vi "ATDome_cancelCallback_command_closeShutterackcmd.vi"(8 "error in (no error)":errorcluster) -> (0 "error out":errorcluster, 3 "function return":i32)   [LabVIEW 2016, in "SALLV_ATDome.lvlib"]
doc: "int ATDome_shm_cancelCallback_command_closeShutter_ackcmdLV();"
uses:
  SALLV_ATDome.lvlib
  SALLV_ATDome.so
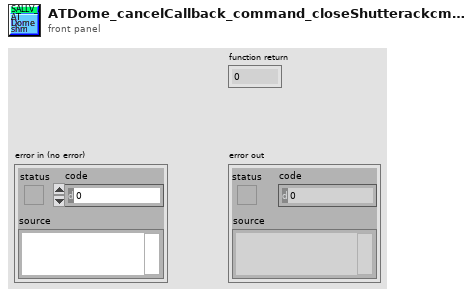
[diagram p1: front panel]
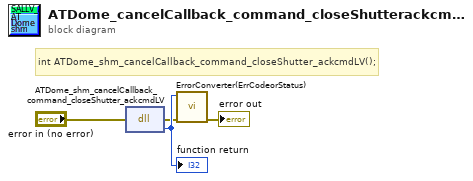
[diagram p0: block diagram]
diagram:
  # "int ATDome_shm_cancelCallback_command_closeShutter_ackcmdLV();"
  n1 = dll-call lib="home/andres/Desktop/SAL_ATDome/SALLV_ATDome.*" fn="ATDome_shm_cancelCallback_command_closeShutter_ackcmdLV"(error in="error in (no error)") -> (error out=w2:errorcluster, w4:i32)  [unwired: 2 in, 1 out]
  "function return" <- w4
  n2 = call "ErrorConverter(ErrCodeorStatus).vi"("error in (no error)"=w2, "error code"=w4) -> ("error out"=→"error out":errorcluster)  [unwired: 9 in]
